vi "Create Status.vi"(8 "error in (no error)":errorcluster, 11 "Framework in":refnum<class "Framework.lvclass">) -> (0 "error out":errorcluster, 3 "Framework out":refnum<class "Framework.lvclass">)   [LabVIEW 2017, in "DSF Core.lvlib" / "Framework.lvclass"]
uses:
  Framework.lvclass
  Framework.lvclass/Framework.ctl
  Status/Framework Status.lvclass
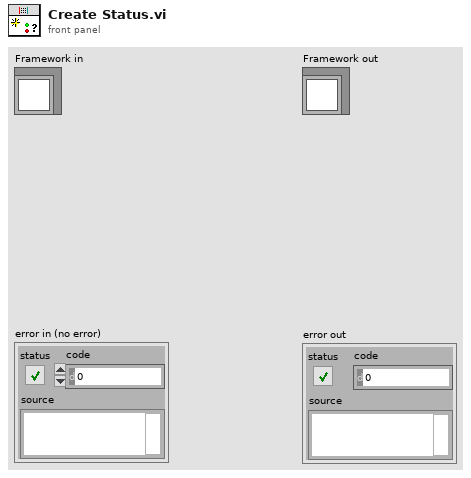
[diagram p1: front panel]
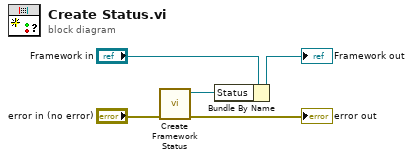
[diagram p0: block diagram]
diagram:
  n1 = call "Create Framework Status.vi"("error in (no error)"="error in (no error)") -> ("error out"=→"error out":errorcluster, "Framework Status"=w2:refnum<class "Framework Status.lvclass">)  [unwired: 9 in]
  n2 = Bundle By Name(cluster="Framework in", "Status"=w2) -> (→"Framework out":refnum<class "Framework.lvclass">)
